vi "Autonomous Independent_17Feb.vi"() -> ()   [LabVIEW 2012]
doc: "This VI is called when autonomous begins, and will automatically be terminated when autonomous ends. You can carry out timed or sensor driven robot movement independently without needing to return to the caller."
uses:
  Robot Global Data.vi
  <vilib>/Rock Robotics/WPI/Joystick/WPI_JoystickGetSetRefNum.vi
  <vilib>/Rock Robotics/WPI/RobotDrive/WPI_RobotDriveArcadeDrive_Standard(NoSaturation).vi
panel:
  out "Prime 3":i32
  out "Prime 2.1":i32
  out "Prime 1.1":i32
  out "Prime 2":i32
  out "Prime 1":i32
  out "Report 2":i32
  out "Report 1":i32
  out "Count 3":bool
  out "Count 2":bool
  out "Count 1":bool
  out "S3":i32
  out "S2":i32
  out "S1":i32
  in  "Auton Pitch":dbl=30.5
  in  "Auton RPM":dbl=4200.0
  in  "milliseconds to wait\nduring autonomous":u32
  in  "Desired angle to\nturn to align with feeder\nstation 2":dbl
  in  "Desired distance for\nencoder to travel straight\ntowards wall 2":dbl
  in  "Desired angle to\nturn towards wall 2":dbl
  in  "Desired distance for\nthe encoder to count 2":dbl
  in  "Desired angle to turn\nBackwards (180) 2":dbl
  in  "Autonomous Modes":T1(ring)
  in  "Desired angle to\nturn to align with feeder\nstation":dbl
  in  "Desired distance for\nencoder to travel straight\ntowards wall":dbl
  in  "Desired angle to\nturn towards wall":dbl
  in  "Desired distance for\nthe encoder to count":dbl
  in  "Desired angle to turn\nBackwards (180)":dbl
  out "Current Movement, for debugging":T2 {"Y Joystick Value" scale=1.0..-1.0; "X Joystick Value" scale=-1.0..1.0}
  in  "Array of robot movements":T3(array[cluster]) {"Y Joystick Value" scale=1.0..-1.0; "X Joystick Value" scale=-1.0..1.0}
  # "Pre-Shot"
  # "Shoot 1"
  # "Shoot 2"
  # "To Align With Protected Feeder Station"
  # "To Align With Unprotected Feeder Station"
  # "Shoot 3"
  # "Be sure to right-click and choose Data Operations>>Make Current Value default if you want to save the array values with the VI"
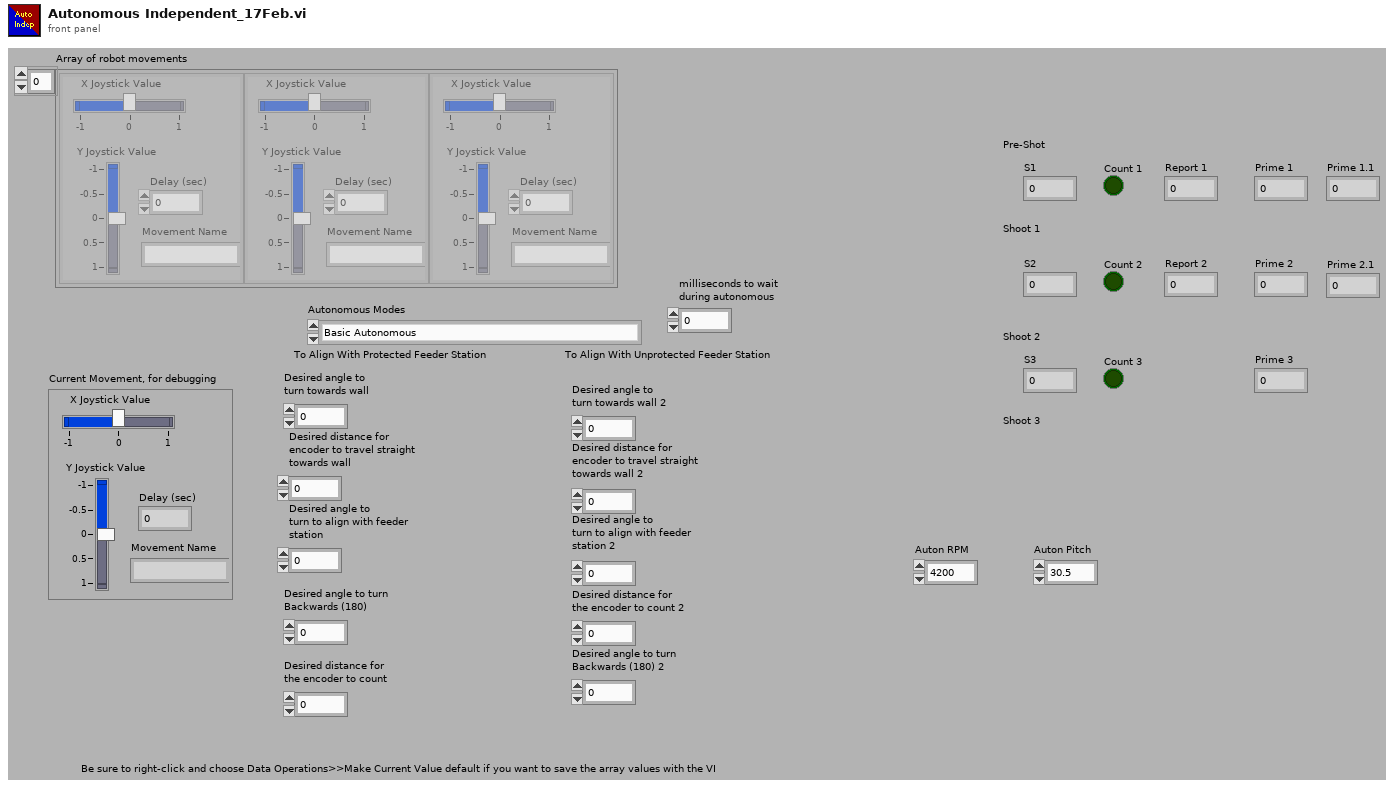
[diagram p1: front panel]
types:
  T1 = enum16{"Basic Autonomous", "Delayed Autonomous", "Shoot and Line Up With Protected Feeder Station", "Shoot and Line Up With Unprotected Feeder Station"}
  T2 = cluster{"X Joystick Value":dbl, "Y Joystick Value":dbl, "Delay (sec)":dbl, "Movement Name":string}
  T3 = cluster{"X Joystick Value":dbl, "Y Joystick Value":dbl, "Delay (sec)":dbl, "Movement Name":string}[]
  T4 = typedef "WPI_JoystickDevRef.ctl" = cluster{"Device":T5}
  T5 = typedef "WPI_JoystickDeviceEnum.ctl" = enum16{"USB 1", "USB 2", "USB 3", "USB 4", "Kinect 1", "Kinect 2"}
  T6 = cluster{"axis 1 (x)":dbl, "axis 2 (y)":dbl, "axis 3 (throttle)":dbl, "axis 4":dbl, "axis 5":dbl, "axis 6":dbl}
  T7 = typedef "WPI_RobotDriveDevRef.ctl" = cluster{"DevStatus":errorcluster, "Motors[]":T8[], "Square Inputs":bool, "Max Output":dbl, "Isochronous":bool}
  T8 = typedef "WPI_MotorControlDeviceRef.ctl" = cluster{"DeviceStatus":errorcluster, "Type":enum16{"PWM", "CAN"}, "PWM":cluster{"Digital Module":T9, "PWM Channel":T10, "DeadBand":T11}, "CAN":cluster{"Device Number":u8, "Control Mode":T12, "Semaphore":T13, "Max Vout":dbl}, "Invert":bool, "TransformRef":T14, "InvTransformRef":T14}
  T9 = typedef "FPGA_TypedefDigitalModule.ctl" = enum16{"Digital Module 1", "Digital Module 2"}
  T10 = typedef "FPGA_DIOPWMChannel.ctl" = enum8{"PWM 1", "PWM 2", "PWM 3", "PWM 4", "PWM 5", "PWM 6", "PWM 7", "PWM 8", "PWM 9", "PWM 10", "Invalid"}
  T11 = typedef "WPI_PWMDeadband.ctl" = cluster{"Name":string, "maxPositivePwm":i32, "minPositivePwm":i32, "centerPwm":i32, "maxNegativePwm":i32, "minNegativePwm":i32, "angularRange":u16}
  T12 = typedef "WPI_CANJaguar_ControlMode.ctl" = enum8{"Percent VBus", "Current", "Speed", "Position", "Voltage"}
  T13 = typedef "Semaphore RefNum" = refnum<k1>
  T14 = typedef "WPI_PWMTransform_ConPane.ctl" = refnum<vi>
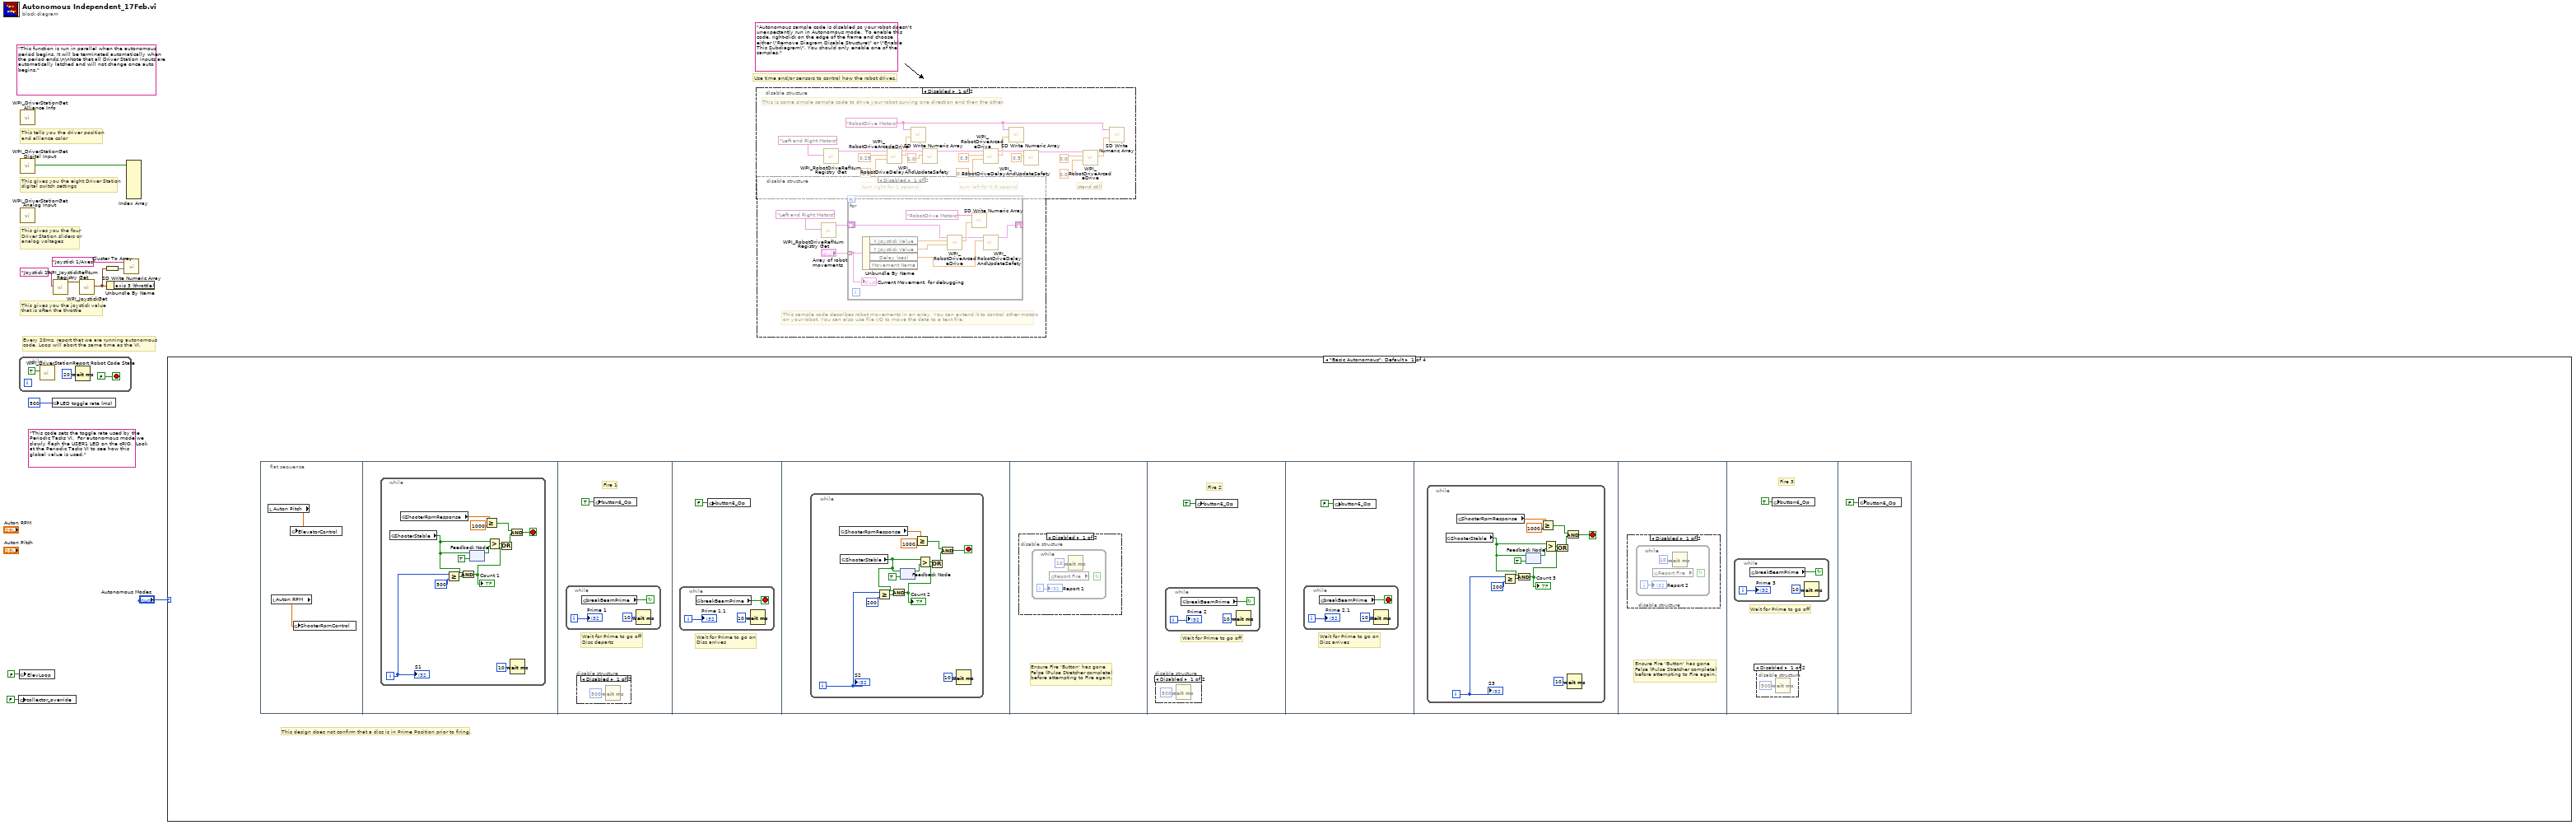
[diagram p0: block diagram]
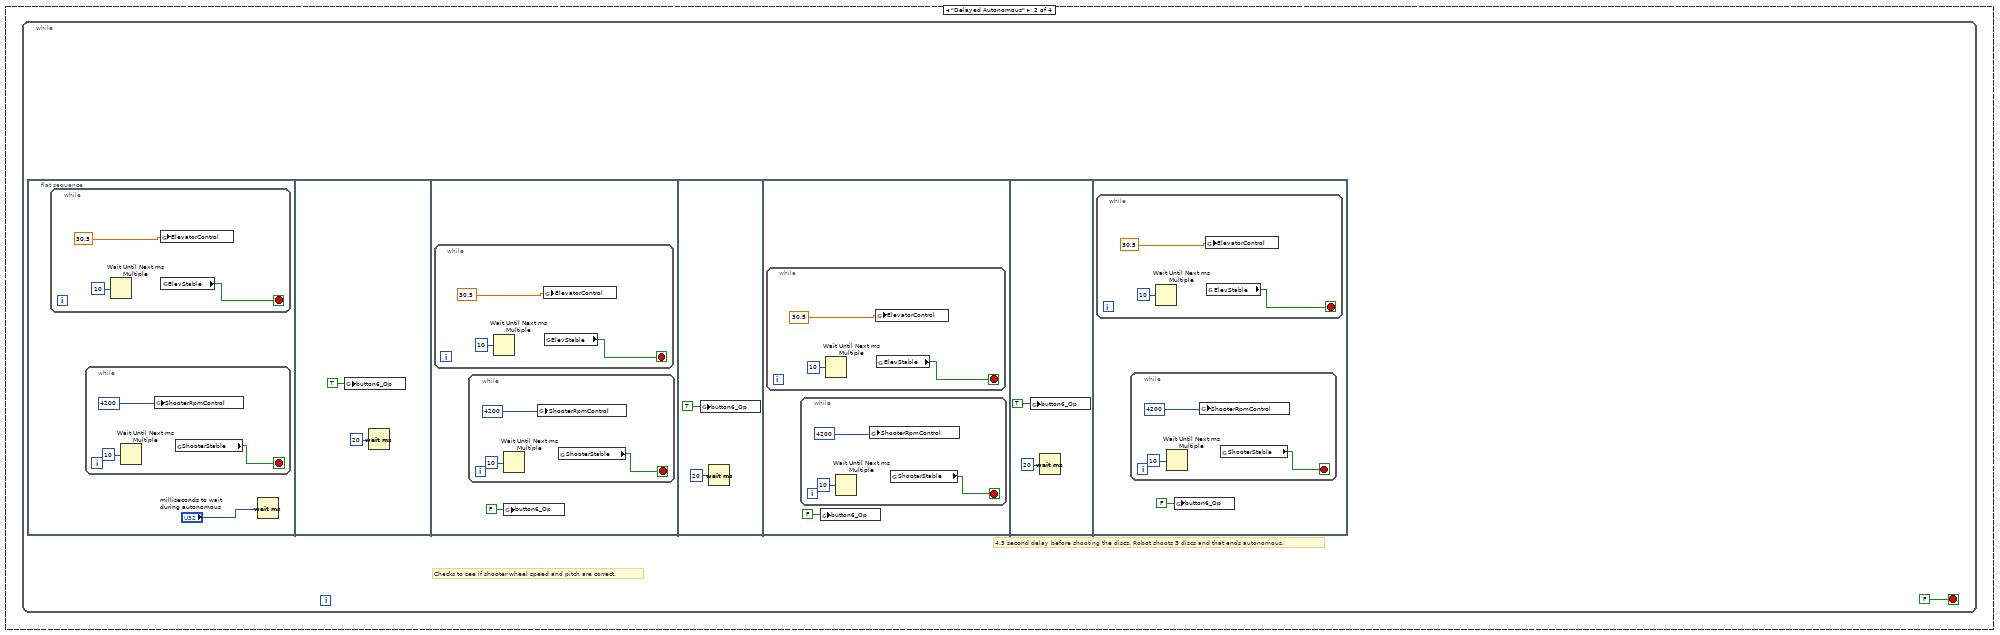
[diagram p7: hidden frame]
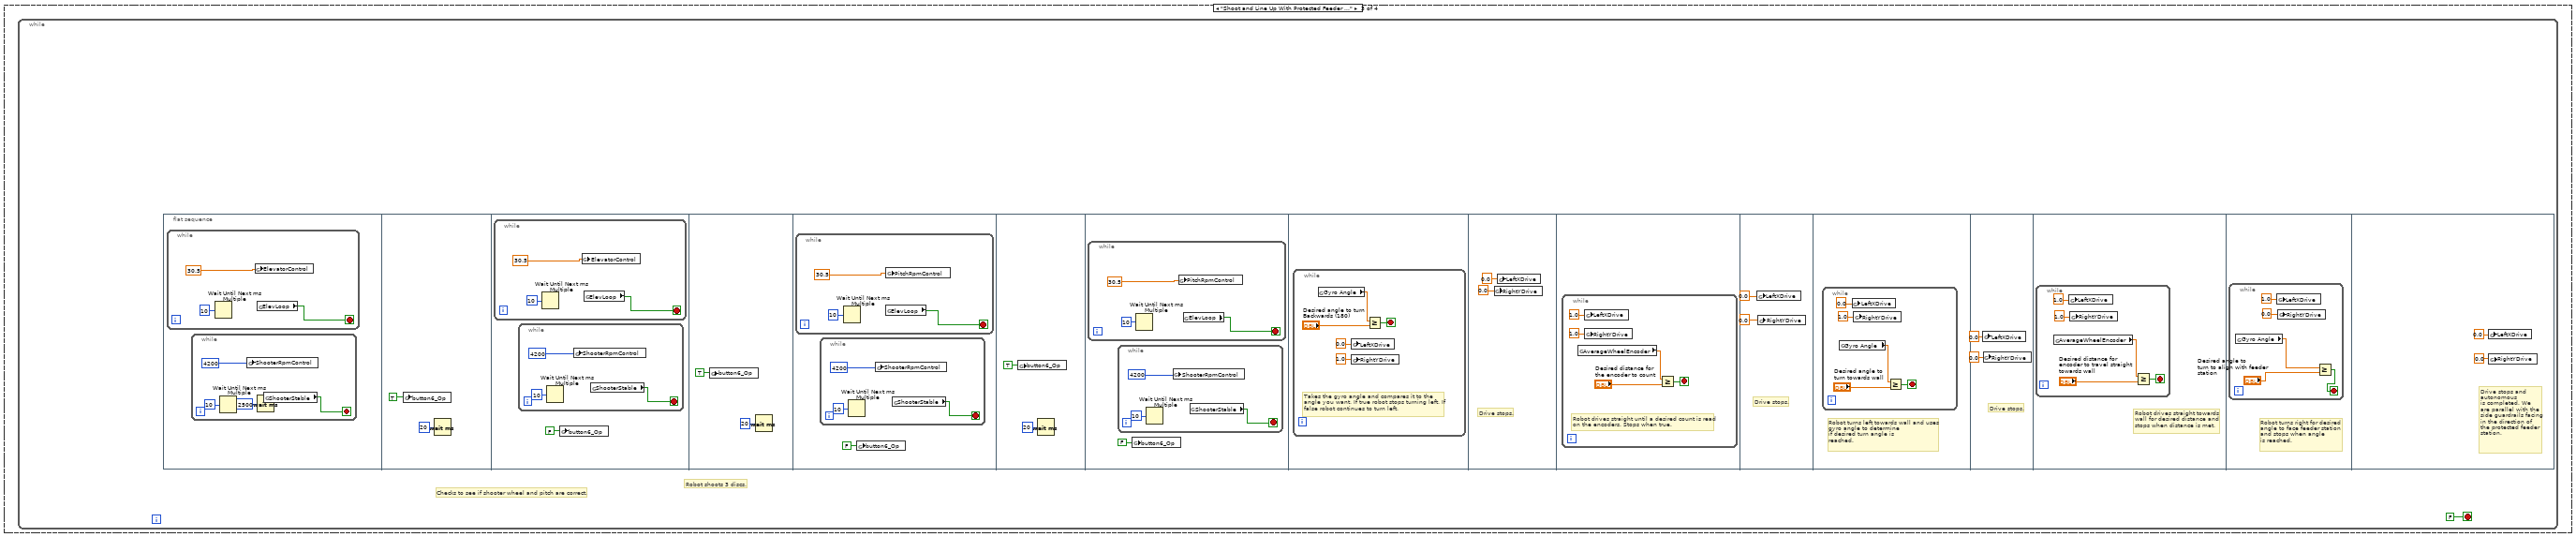
[diagram p8: hidden frame]
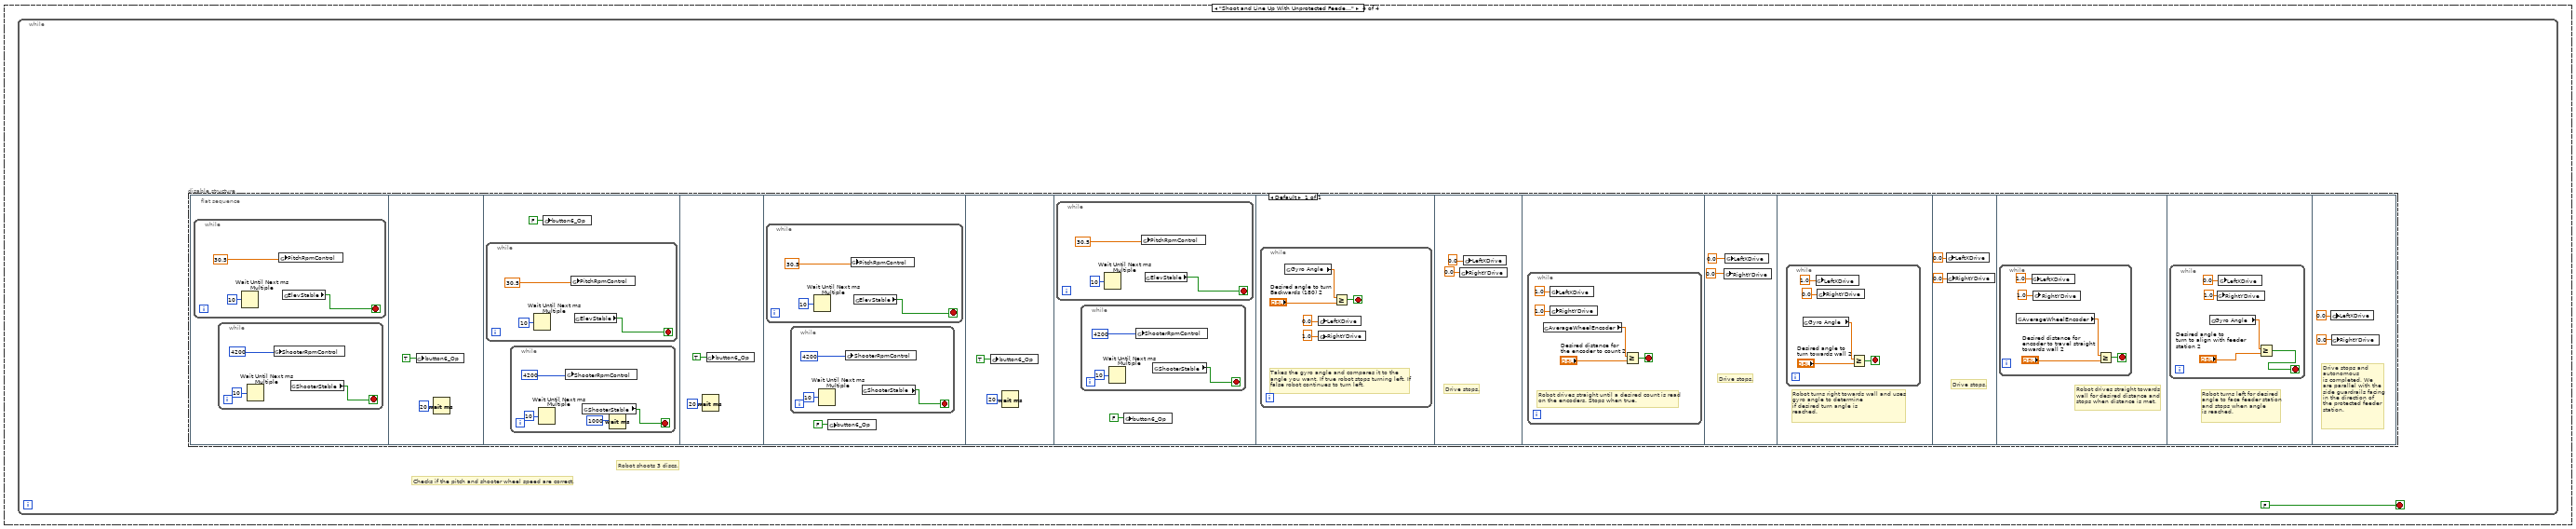
[diagram p9: hidden frame]
diagram:
  (unwired) "This code sets the toggle rate used by the Periodic Tasks VI.  For autonomous mode we slowly flash the USER1 LED on the cRIO.  Look at the Periodic Tasks VI to see how this global value is used."
  (unwired) "Autonomous sample code is disabled so your robot doesn't unexpectantly run in Autonomous mode.  To enable this code, right-click on the edge of the frame and choose either \"Remove Diagram Disable Structure\" or \"Enable This Subdiagram\". You should only enable one of the samples."
  (unwired) "This function is run in parallel when the autonomous period begins. It will be terminated automatically when the period ends.\n\nNote that all Driver Station inputs are automatically latched and will not change once auto begins."
  # "Every 20ms, report that we are running autonomous\ncode. Loop will abort the same time as the VI."
  # "This gives you the joystick value\nthat is often the throttle"
  # "Use time and/or sensors to control how the robot drives."
  # "This tells you the driver position\nand alliance color"
  # "This gives you the eight Driver Station\ndigital switch settings"
  # "This gives you the four\nDriver Station sliders or\nanalog voltages"
  n1 = global write "Robot Global Data.vi" "collector_override"(FALSE ("collector_override")) -> ()
  n2 = global write "Robot Global Data.vi" "ElevLoop"(FALSE ("ElevLoop")) -> ()
  n3 = while {
    stop <- FALSE stop-if-true
    n4 = call <vilib>:"WPI_DriverStationReport Robot Code State.vi"("Autonomous"=TRUE) -> ()  [unwired: 10 in, 1 out]
    n5 = Wait (ms)(milliseconds to wait=u32 20) -> ()  [unwired: 1 out]
  }
  n6 = call <vilib>:"WPI_DriverStationGet Alliance Info.vi"() -> ()  [unwired: 12 out]
  n7 = call <vilib>:"WPI_DriverStationGet Digital Input.vi"() -> ("Driver Station Digital Input (1-8)"=w10:bool[])  [unwired: 11 out]
  n8 = call <vilib>:"WPI_DriverStationGet Analog Input.vi"() -> ()  [unwired: 12 out]
  n9 = global write "Robot Global Data.vi" "LED toggle rate (ms)"(u32 500 ("LED ms toggle rate")) -> ()
  n10 = call <vilib>:"WPI_JoystickRefNum Registry Get.vi"("refnum name"="Joystick 1") -> ("JoystickDevRef"=w8:T4)  [unwired: 1 in, 9 out]
  n11 = call <vilib>:"WPI_JoystickGet.vi"("JoystickDevRef"=w8) -> ("Axes"=w5:T6)  [unwired: 1 in, 5 out]
  n12 = Cluster To Array(cluster=w5) -> (array=w6:dbl[])
  n13 = Unbundle By Name(w5) -> ()  [unwired: 1 out]
  n14 = call <vilib>:"SD Write Numeric Array.vi"("Numeric Array"=w6, "Name"="Joystick 1/Axes") -> ()  [unwired: 8 in, 2 out]
  n15 = Index Array(array=w10) -> ()  [unwired: 8 in, 8 out]
  n16 = case shown="\"Basic Autonomous\", Default" "Autonomous Modes" {
    frame "Basic Autonomous", Default {
      # "This design does not confirm that a disc is in Prime Position prior to firing."
      n17 = flat-sequence {
        frame #0 {
          n18 = local read "Auton Pitch"() -> (w15:dbl)
          n19 = local read "Auton RPM"() -> (w14:dbl)
          n20 = global write "Robot Global Data.vi" "ElevatorControl"(w15) -> ()
          n21 = global write "Robot Global Data.vi" "ShooterRpmControl"(w14) -> ()
        }
        frame #1 {
          n22 = while {
            i -> [w18]
            stop <- w16 stop-if-true
            n23 = global read "Robot Global Data.vi" "ShooterStable"() -> (w17:bool)
            n24 = global read "Robot Global Data.vi" "ShooterRpmResponse"() -> (w19:dbl)
            n25 = Greater Or Equal?(x=w18, y=500) -> (x >= y?=w24:bool)
            n26 = And(x=w17, y=w24) -> (x .and. y?=w26:bool)
            "Count 1" <- w26
            n27 = feedback #1(TRUE ("Shooter Stable?")) -> (w22:bool)
            n28 = feedback-in #1(w17) -> ()
            n29 = Greater Or Equal?(x=w19, y=1000.0) -> (x >= y?=w21:bool)
            n30 = Greater?(x=w17, y=w22) -> (0:w27:bool)
            n31 = Or(x=w27, y=w26) -> (x .or. y?=w28:bool)
            n32 = And(x=w21, y=w28) -> (x .and. y?=w16:bool)
            n33 = Wait (ms)(milliseconds to wait=u32 10 ("millisecond multiple")) -> ()  [unwired: 1 out]
            "S1" <- w18
          }
        }
        frame #2 {
          # "Wait for Prime to go off\nDisc departs"
          # "Fire 1"
          n34 = while {
            i -> [w32]
            stop <- w34 continue-if-true
            n35 = global read "Robot Global Data.vi" "breakBeamPrime"() -> (w34:bool)
            n36 = Wait (ms)(milliseconds to wait=u32 10 ("millisecond multiple")) -> ()  [unwired: 1 out]
            "Prime 1" <- w32
          }
          n37 = disable-structure shown="Disabled" {
            frame Disabled {
              n38 = Wait (ms)(milliseconds to wait=u32 500) -> ()  [unwired: 1 out]
            }
            frame Enabled {
            }
          }
          n39 = global write "Robot Global Data.vi" "button6_Op"(TRUE ("button5_Op")) -> ()
        }
        frame #3 {
          # "Wait for Prime to go on\nDisc arrives"
          n40 = while {
            i -> [w36]
            stop <- w38 stop-if-true
            n41 = global read "Robot Global Data.vi" "breakBeamPrime"() -> (w38:bool)
            n42 = Wait (ms)(milliseconds to wait=u32 10 ("millisecond multiple")) -> ()  [unwired: 1 out]
            "Prime 1.1" <- w36
          }
          n43 = global write "Robot Global Data.vi" "button6_Op"(FALSE ("button5_Op")) -> ()
        }
        frame #4 {
          n44 = while {
            i -> [w40]
            stop <- w39 stop-if-true
            n45 = global read "Robot Global Data.vi" "ShooterRpmResponse"() -> (w51:dbl)
            n46 = global read "Robot Global Data.vi" "ShooterStable"() -> (w43:bool)
            n47 = Greater Or Equal?(x=w40, y=200) -> (x >= y?=w46:bool)
            n48 = And(x=w43, y=w46) -> (x .and. y?=w44:bool)
            "Count 2" <- w44
            n49 = feedback #2(TRUE ("Shooter Stable?")) -> (w48:bool)
            n50 = feedback-in #2(w43) -> ()
            n51 = Greater Or Equal?(x=w51, y=1000.0) -> (x >= y?=w49:bool)
            n52 = Greater?(x=w43, y=w48) -> (0:w42:bool)
            n53 = Or(x=w42, y=w44) -> (x .or. y?=w41:bool)
            n54 = And(x=w49, y=w41) -> (x .and. y?=w39:bool)
            n55 = Wait (ms)(milliseconds to wait=u32 10 ("millisecond multiple")) -> ()  [unwired: 1 out]
            "S2" <- w40
          }
        }
        frame #5 {
          # "Ensure Fire 'Button' has gone\nFalse (Pulse Stretcher complete)\nbefore attempting to Fire again."
          n56 = disable-structure shown="Disabled" {
            frame Disabled {
              n57 = while {
                i -> [w54]
                stop <- _ continue-if-true
                n58 = global read "Robot Global Data.vi" "Report Fire"() -> ()  [unwired: 1 out]
                n59 = Wait (ms)(milliseconds to wait=u32 10) -> ()  [unwired: 1 out]
                "Report 1" <- w54
              }
            }
            frame Enabled {
            }
          }
        }
        frame #6 {
          # "Wait for Prime to go off"
          # "Fire 2"
          n60 = disable-structure shown="Disabled" {
            frame Disabled {
              n61 = Wait (ms)(milliseconds to wait=u32 500) -> ()  [unwired: 1 out]
            }
            frame Enabled {
            }
          }
          n62 = while {
            i -> [w56]
            stop <- w58 continue-if-true
            n63 = global read "Robot Global Data.vi" "breakBeamPrime"() -> (w58:bool)
            n64 = Wait (ms)(milliseconds to wait=u32 10 ("millisecond multiple")) -> ()  [unwired: 1 out]
            "Prime 2" <- w56
          }
          n65 = global write "Robot Global Data.vi" "button6_Op"(TRUE ("button5_Op")) -> ()
        }
        frame #7 {
          # "Wait for Prime to go on\nDisc arrives"
          n66 = while {
            i -> [w61]
            stop <- w63 stop-if-true
            n67 = global read "Robot Global Data.vi" "breakBeamPrime"() -> (w63:bool)
            n68 = Wait (ms)(milliseconds to wait=u32 10 ("millisecond multiple")) -> ()  [unwired: 1 out]
            "Prime 2.1" <- w61
          }
          n69 = global write "Robot Global Data.vi" "button6_Op"(FALSE ("button5_Op")) -> ()
        }
        frame #8 {
          n70 = while {
            i -> [w65]
            stop <- w64 stop-if-true
            n71 = global read "Robot Global Data.vi" "ShooterStable"() -> (w66:bool)
            n72 = global read "Robot Global Data.vi" "ShooterRpmResponse"() -> (w67:dbl)
            n73 = Greater Or Equal?(x=w65, y=200) -> (x >= y?=w72:bool)
            n74 = And(x=w66, y=w72) -> (x .and. y?=w74:bool)
            "Count 3" <- w74
            n75 = feedback #3(TRUE ("Shooter Stable?")) -> (w70:bool)
            n76 = feedback-in #3(w66) -> ()
            n77 = Greater Or Equal?(x=w67, y=1000.0) -> (x >= y?=w69:bool)
            n78 = Greater?(x=w66, y=w70) -> (0:w75:bool)
            n79 = Or(x=w75, y=w74) -> (x .or. y?=w76:bool)
            n80 = And(x=w69, y=w76) -> (x .and. y?=w64:bool)
            n81 = Wait (ms)(milliseconds to wait=u32 10 ("millisecond multiple")) -> ()  [unwired: 1 out]
            "S3" <- w65
          }
        }
        frame #9 {
          # "Ensure Fire 'Button' has gone\nFalse (Pulse Stretcher complete)\nbefore attempting to Fire again."
          n82 = disable-structure shown="Disabled" {
            frame Disabled {
              n83 = while {
                i -> [w79]
                stop <- _ continue-if-true
                n84 = global read "Robot Global Data.vi" "Report Fire"() -> ()  [unwired: 1 out]
                n85 = Wait (ms)(milliseconds to wait=u32 10) -> ()  [unwired: 1 out]
                "Report 2" <- w79
              }
            }
            frame Enabled {
            }
          }
        }
        frame #10 {
          # "Wait for Prime to go off"
          # "Fire 3"
          n86 = while {
            i -> [w81]
            stop <- w83 continue-if-true
            n87 = global read "Robot Global Data.vi" "breakBeamPrime"() -> (w83:bool)
            n88 = Wait (ms)(milliseconds to wait=u32 10 ("millisecond multiple")) -> ()  [unwired: 1 out]
            "Prime 3" <- w81
          }
          n89 = disable-structure shown="Disabled" {
            frame Disabled {
              n90 = Wait (ms)(milliseconds to wait=u32 500) -> ()  [unwired: 1 out]
            }
            frame Enabled {
            }
          }
          n91 = global write "Robot Global Data.vi" "button6_Op"(TRUE ("button5_Op")) -> ()
        }
        frame #11 {
          n92 = global write "Robot Global Data.vi" "button6_Op"(FALSE ("button5_Op")) -> ()
        }
      }
    }
    frame "Delayed Autonomous" {
      n93 = while {
        stop <- FALSE stop-if-true
        # "Checks to see if shooter wheel speed and pitch are correct."
        # "4.5 second delay before shooting the discs. Robot shoots 3 discs and that ends autonomous."
        n94 = flat-sequence {
          frame #0 {
            n95 = while {
              stop <- w89 stop-if-true
              n96 = Wait Until Next ms Multiple(millisecond multiple=u32 10) -> ()  [unwired: 1 out]
              n97 = global write "Robot Global Data.vi" "ElevatorControl"(30.5 ("y")) -> ()
              n98 = global read "Robot Global Data.vi" "ElevStable"() -> (w89:bool)
            }
            n99 = while {
              stop <- w92 stop-if-true
              n100 = Wait Until Next ms Multiple(millisecond multiple=u32 10) -> ()  [unwired: 1 out]
              n101 = global write "Robot Global Data.vi" "ShooterRpmControl"(4200 ("Value")) -> ()
              n102 = global read "Robot Global Data.vi" "ShooterStable"() -> (w92:bool)
            }
            n103 = Wait (ms)(milliseconds to wait="milliseconds to wait\nduring autonomous") -> ()  [unwired: 1 out]
          }
          frame #1 {
            n104 = global write "Robot Global Data.vi" "button6_Op"(TRUE ("button5_Op")) -> ()
            n105 = Wait (ms)(milliseconds to wait=u32 20) -> ()  [unwired: 1 out]
          }
          frame #2 {
            n106 = while {
              stop <- w98 stop-if-true
              n107 = Wait Until Next ms Multiple(millisecond multiple=u32 10) -> ()  [unwired: 1 out]
              n108 = global write "Robot Global Data.vi" "ElevatorControl"(30.5 ("y")) -> ()
              n109 = global read "Robot Global Data.vi" "ElevStable"() -> (w98:bool)
            }
            n110 = while {
              stop <- w101 stop-if-true
              n111 = Wait Until Next ms Multiple(millisecond multiple=u32 10) -> ()  [unwired: 1 out]
              n112 = global write "Robot Global Data.vi" "ShooterRpmControl"(4200 ("Value")) -> ()
              n113 = global read "Robot Global Data.vi" "ShooterStable"() -> (w101:bool)
            }
            n114 = global write "Robot Global Data.vi" "button6_Op"(FALSE ("button5_Op")) -> ()
          }
          frame #3 {
            n115 = global write "Robot Global Data.vi" "button6_Op"(TRUE ("button5_Op")) -> ()
            n116 = Wait (ms)(milliseconds to wait=u32 20) -> ()  [unwired: 1 out]
          }
          frame #4 {
            n117 = while {
              stop <- w107 stop-if-true
              n118 = Wait Until Next ms Multiple(millisecond multiple=u32 10) -> ()  [unwired: 1 out]
              n119 = global write "Robot Global Data.vi" "ElevatorControl"(30.5 ("y")) -> ()
              n120 = global read "Robot Global Data.vi" "ElevStable"() -> (w107:bool)
            }
            n121 = while {
              stop <- w110 stop-if-true
              n122 = Wait Until Next ms Multiple(millisecond multiple=u32 10) -> ()  [unwired: 1 out]
              n123 = global write "Robot Global Data.vi" "ShooterRpmControl"(4200 ("Value")) -> ()
              n124 = global read "Robot Global Data.vi" "ShooterStable"() -> (w110:bool)
            }
            n125 = global write "Robot Global Data.vi" "button6_Op"(FALSE ("button5_Op")) -> ()
          }
          frame #5 {
            n126 = global write "Robot Global Data.vi" "button6_Op"(TRUE ("button5_Op")) -> ()
            n127 = Wait (ms)(milliseconds to wait=u32 20) -> ()  [unwired: 1 out]
          }
          frame #6 {
            n128 = while {
              stop <- w116 stop-if-true
              n129 = Wait Until Next ms Multiple(millisecond multiple=u32 10) -> ()  [unwired: 1 out]
              n130 = global write "Robot Global Data.vi" "ElevatorControl"(30.5 ("y")) -> ()
              n131 = global read "Robot Global Data.vi" "ElevStable"() -> (w116:bool)
            }
            n132 = while {
              stop <- w119 stop-if-true
              n133 = Wait Until Next ms Multiple(millisecond multiple=u32 10) -> ()  [unwired: 1 out]
              n134 = global write "Robot Global Data.vi" "ShooterRpmControl"(4200 ("Value")) -> ()
              n135 = global read "Robot Global Data.vi" "ShooterStable"() -> (w119:bool)
            }
            n136 = global write "Robot Global Data.vi" "button6_Op"(FALSE ("button5_Op")) -> ()
          }
        }
      }
    }
    frame "Shoot and Line Up With Protected Feeder Station" {
      n137 = while {
        stop <- FALSE stop-if-true
        # "Checks to see if shooter wheel and pitch are correct."
        # "Robot shoots 3 discs."
        n138 = flat-sequence {
          frame #0 {
            n139 = while {
              stop <- w124 stop-if-true
              n140 = Wait Until Next ms Multiple(millisecond multiple=u32 10) -> ()  [unwired: 1 out]
              n141 = global write "Robot Global Data.vi" "ElevatorControl"(30.5 ("y")) -> ()
              n142 = global read "Robot Global Data.vi" "ElevLoop"() -> (w124:bool)
            }
            n143 = while {
              stop <- w127 stop-if-true
              n144 = Wait Until Next ms Multiple(millisecond multiple=u32 10) -> ()  [unwired: 1 out]
              n145 = global write "Robot Global Data.vi" "ShooterRpmControl"(4200 ("Value")) -> ()
              n146 = global read "Robot Global Data.vi" "ShooterStable"() -> (w127:bool)
            }
            n147 = Wait (ms)(milliseconds to wait=u32 2500) -> ()  [unwired: 1 out]
          }
          frame #1 {
            n148 = global write "Robot Global Data.vi" "button6_Op"(TRUE ("button5_Op")) -> ()
            n149 = Wait (ms)(milliseconds to wait=u32 20) -> ()  [unwired: 1 out]
          }
          frame #2 {
            n150 = while {
              stop <- w133 stop-if-true
              n151 = Wait Until Next ms Multiple(millisecond multiple=u32 10) -> ()  [unwired: 1 out]
              n152 = global write "Robot Global Data.vi" "ElevatorControl"(30.5 ("y")) -> ()
              n153 = global read "Robot Global Data.vi" "ElevLoop"() -> (w133:bool)
            }
            n154 = while {
              stop <- w136 stop-if-true
              n155 = Wait Until Next ms Multiple(millisecond multiple=u32 10) -> ()  [unwired: 1 out]
              n156 = global write "Robot Global Data.vi" "ShooterRpmControl"(4200 ("Value")) -> ()
              n157 = global read "Robot Global Data.vi" "ShooterStable"() -> (w136:bool)
            }
            n158 = global write "Robot Global Data.vi" "button6_Op"(FALSE ("button5_Op")) -> ()
          }
          frame #3 {
            n159 = global write "Robot Global Data.vi" "button6_Op"(TRUE ("button5_Op")) -> ()
            n160 = Wait (ms)(milliseconds to wait=u32 20) -> ()  [unwired: 1 out]
          }
          frame #4 {
            n161 = while {
              stop <- w142 stop-if-true
              n162 = Wait Until Next ms Multiple(millisecond multiple=u32 10) -> ()  [unwired: 1 out]
              n163 = global read "Robot Global Data.vi" "ElevLoop"() -> (w142:bool)
              n164 = global write "Robot Global Data.vi" "PitchRpmControl"(30.5 ("y")) -> ()
            }
            n165 = while {
              stop <- w145 stop-if-true
              n166 = Wait Until Next ms Multiple(millisecond multiple=u32 10) -> ()  [unwired: 1 out]
              n167 = global write "Robot Global Data.vi" "ShooterRpmControl"(4200 ("Value")) -> ()
              n168 = global read "Robot Global Data.vi" "ShooterStable"() -> (w145:bool)
            }
            n169 = global write "Robot Global Data.vi" "button6_Op"(FALSE ("button5_Op")) -> ()
          }
          frame #5 {
            n170 = global write "Robot Global Data.vi" "button6_Op"(TRUE ("button5_Op")) -> ()
            n171 = Wait (ms)(milliseconds to wait=u32 20) -> ()  [unwired: 1 out]
          }
          frame #6 {
            n172 = while {
              stop <- w151 stop-if-true
              n173 = Wait Until Next ms Multiple(millisecond multiple=u32 10) -> ()  [unwired: 1 out]
              n174 = global write "Robot Global Data.vi" "PitchRpmControl"(30.5 ("y")) -> ()
              n175 = global read "Robot Global Data.vi" "ElevLoop"() -> (w151:bool)
            }
            n176 = while {
              stop <- w154 stop-if-true
              n177 = Wait Until Next ms Multiple(millisecond multiple=u32 10) -> ()  [unwired: 1 out]
              n178 = global write "Robot Global Data.vi" "ShooterRpmControl"(4200 ("Value")) -> ()
              n179 = global read "Robot Global Data.vi" "ShooterStable"() -> (w154:bool)
            }
            n180 = global write "Robot Global Data.vi" "button6_Op"(FALSE ("button5_Op")) -> ()
          }
          frame #7 {
            n181 = while {
              stop <- w160 stop-if-true
              # "Takes the gyro angle and compares it to the\nangle you want. If true robot stops turning left. If\nfalse robot continues to turn left."
              n182 = global read "Robot Global Data.vi" "Gyro Angle"() -> (w156:dbl)
              n183 = global write "Robot Global Data.vi" "LeftXDrive"(0.0 ("Left axis value")) -> ()
              n184 = global write "Robot Global Data.vi" "RightYDrive"(1.0 ("Right axis value")) -> ()
              n185 = Greater Or Equal?(x=w156, y="Desired angle to turn\nBackwards (180)") -> (x >= y?=w160:bool)
            }
          }
          frame #8 {
            # "Drive stops."
            n186 = global write "Robot Global Data.vi" "RightYDrive"(0.0 ("Right axis value")) -> ()
            n187 = global write "Robot Global Data.vi" "LeftXDrive"(0.0 ("Left axis value")) -> ()
          }
          frame #9 {
            n188 = while {
              stop <- w165 stop-if-true
              # "Robot drives straight until a desired count is read\non the encoders. Stops when true."
              n189 = global read "Robot Global Data.vi" "AverageWheelEncoder"() -> (w167:dbl)
              n190 = global write "Robot Global Data.vi" "LeftXDrive"(1.0 ("Left axis value")) -> ()
              n191 = global write "Robot Global Data.vi" "RightYDrive"(1.0 ("Right axis value")) -> ()
              n192 = Greater Or Equal?(x=w167, y="Desired distance for\nthe encoder to count") -> (x >= y?=w165:bool)
            }
          }
          frame #10 {
            # "Drive stops."
            n193 = global write "Robot Global Data.vi" "LeftXDrive"(0.0 ("LeftXDrive")) -> ()
            n194 = global write "Robot Global Data.vi" "RightYDrive"(0.0 ("LeftXDrive")) -> ()
          }
          frame #11 {
            # "Robot turns left towards wall and uses\ngyro angle to determine\nif desired turn angle is \nreached."
            n195 = while {
              stop <- w171 stop-if-true
              n196 = global read "Robot Global Data.vi" "Gyro Angle"() -> (w170:dbl)
              n197 = global write "Robot Global Data.vi" "LeftXDrive"(0.0 ("Left axis value")) -> ()
              n198 = global write "Robot Global Data.vi" "RightYDrive"(1.0 ("Right axis value")) -> ()
              n199 = Greater Or Equal?(x=w170, y="Desired angle to\nturn towards wall") -> (x >= y?=w171:bool)
            }
          }
          frame #12 {
            # "Drive stops."
            n200 = global write "Robot Global Data.vi" "LeftXDrive"(0.0 ("LeftXDrive")) -> ()
            n201 = global write "Robot Global Data.vi" "RightYDrive"(0.0 ("RightYDrive")) -> ()
          }
          frame #13 {
            # "Robot drives straight towards\nwall for desired distance and\nstops when distance is met."
            n202 = while {
              stop <- w177 stop-if-true
              n203 = global read "Robot Global Data.vi" "AverageWheelEncoder"() -> (w179:dbl)
              n204 = global write "Robot Global Data.vi" "LeftXDrive"(1.0 ("Left axis value")) -> ()
              n205 = global write "Robot Global Data.vi" "RightYDrive"(1.0 ("Right axis value")) -> ()
              n206 = Greater Or Equal?(x=w179, y="Desired distance for\nencoder to travel straight\ntowards wall") -> (x >= y?=w177:bool)
            }
          }
          frame #14 {
            # "Robot turns right for desired\nangle to face feeder station\nand stops when angle\nis reached."
            n207 = while {
              stop <- w183 stop-if-true
              n208 = global read "Robot Global Data.vi" "Gyro Angle"() -> (w182:dbl)
              n209 = global write "Robot Global Data.vi" "LeftXDrive"(1.0 ("Left axis value")) -> ()
              n210 = global write "Robot Global Data.vi" "RightYDrive"(0.0 ("Right axis value")) -> ()
              n211 = Greater Or Equal?(x=w182, y="Desired angle to\nturn to align with feeder\nstation") -> (x >= y?=w183:bool)
            }
          }
          frame #15 {
            # "Drive stops and\nautonomous\nis completed. We\nare parallel with the\nside guardrails facing\nin the direction of\nthe protected feeder\nstation."
            n212 = global write "Robot Global Data.vi" "LeftXDrive"(0.0 ("LeftXDrive")) -> ()
            n213 = global write "Robot Global Data.vi" "RightYDrive"(0.0 ("LeftXDrive")) -> ()
          }
        }
      }
    }
    frame "Shoot and Line Up With Unprotected Feeder Station" {
      n214 = while {
        stop <- FALSE stop-if-true
        # "Checks if the pitch and shooter wheel speed are correct."
        # "Robot shoots 3 discs."
        n215 = disable-structure shown="Default" {
          frame Enabled {
            n216 = flat-sequence {
              frame #0 {
                n217 = while {
                  stop <- w191 stop-if-true
                  n218 = Wait Until Next ms Multiple(millisecond multiple=u32 10) -> ()  [unwired: 1 out]
                  n219 = global write "Robot Global Data.vi" "PitchRpmControl"(30.5 ("y")) -> ()
                  n220 = global read "Robot Global Data.vi" "ElevStable"() -> (w191:bool)
                }
                n221 = while {
                  stop <- w194 stop-if-true
                  n222 = Wait Until Next ms Multiple(millisecond multiple=u32 10) -> ()  [unwired: 1 out]
                  n223 = global write "Robot Global Data.vi" "ShooterRpmControl"(4200 ("Value")) -> ()
                  n224 = global read "Robot Global Data.vi" "ShooterStable"() -> (w194:bool)
                }
              }
              frame #1 {
                n225 = global write "Robot Global Data.vi" "button6_Op"(TRUE ("button5_Op")) -> ()
                n226 = Wait (ms)(milliseconds to wait=u32 20) -> ()  [unwired: 1 out]
              }
              frame #2 {
                n227 = while {
                  stop <- w201 stop-if-true
                  n228 = Wait Until Next ms Multiple(millisecond multiple=u32 10) -> ()  [unwired: 1 out]
                  n229 = global write "Robot Global Data.vi" "PitchRpmControl"(30.5 ("y")) -> ()
                  n230 = global read "Robot Global Data.vi" "ElevStable"() -> (w201:bool)
                }
                n231 = while {
                  stop <- w204 stop-if-true
                  n232 = Wait Until Next ms Multiple(millisecond multiple=u32 10) -> ()  [unwired: 1 out]
                  n233 = global write "Robot Global Data.vi" "ShooterRpmControl"(4200 ("Value")) -> ()
                  n234 = global read "Robot Global Data.vi" "ShooterStable"() -> (w204:bool)
                }
                n235 = global write "Robot Global Data.vi" "button6_Op"(FALSE ("button5_Op")) -> ()
                n236 = Wait (ms)(milliseconds to wait=u32 1000) -> ()  [unwired: 1 out]
              }
              frame #3 {
                n237 = Wait (ms)(milliseconds to wait=u32 20) -> ()  [unwired: 1 out]
                n238 = global write "Robot Global Data.vi" "button6_Op"(TRUE ("button5_Op")) -> ()
              }
              frame #4 {
                n239 = while {
                  stop <- w210 stop-if-true
                  n240 = Wait Until Next ms Multiple(millisecond multiple=u32 10) -> ()  [unwired: 1 out]
                  n241 = global write "Robot Global Data.vi" "PitchRpmControl"(30.5 ("y")) -> ()
                  n242 = global read "Robot Global Data.vi" "ElevStable"() -> (w210:bool)
                }
                n243 = while {
                  stop <- w213 stop-if-true
                  n244 = Wait Until Next ms Multiple(millisecond multiple=u32 10) -> ()  [unwired: 1 out]
                  n245 = global write "Robot Global Data.vi" "ShooterRpmControl"(4200 ("Value")) -> ()
                  n246 = global read "Robot Global Data.vi" "ShooterStable"() -> (w213:bool)
                }
                n247 = global write "Robot Global Data.vi" "button6_Op"(FALSE ("button5_Op")) -> ()
              }
              frame #5 {
                n248 = global write "Robot Global Data.vi" "button6_Op"(TRUE ("button5_Op")) -> ()
                n249 = Wait (ms)(milliseconds to wait=u32 20) -> ()  [unwired: 1 out]
              }
              frame #6 {
                n250 = while {
                  stop <- w219 stop-if-true
                  n251 = Wait Until Next ms Multiple(millisecond multiple=u32 10) -> ()  [unwired: 1 out]
                  n252 = global write "Robot Global Data.vi" "PitchRpmControl"(30.5 ("y")) -> ()
                  n253 = global read "Robot Global Data.vi" "ElevStable"() -> (w219:bool)
                }
                n254 = while {
                  stop <- w222 stop-if-true
                  n255 = Wait Until Next ms Multiple(millisecond multiple=u32 10) -> ()  [unwired: 1 out]
                  n256 = global write "Robot Global Data.vi" "ShooterRpmControl"(4200 ("Value")) -> ()
                  n257 = global read "Robot Global Data.vi" "ShooterStable"() -> (w222:bool)
                }
                n258 = global write "Robot Global Data.vi" "button6_Op"(FALSE ("button5_Op")) -> ()
              }
              frame #7 {
                n259 = while {
                  stop <- w228 stop-if-true
                  # "Takes the gyro angle and compares it to the\nangle you want. If true robot stops turning left. If\nfalse robot continues to turn left."
                  n260 = global read "Robot Global Data.vi" "Gyro Angle"() -> (w224:dbl)
                  n261 = global write "Robot Global Data.vi" "LeftXDrive"(0.0 ("Left axis value")) -> ()
                  n262 = global write "Robot Global Data.vi" "RightYDrive"(1.0 ("Right axis value")) -> ()
                  n263 = Greater Or Equal?(x=w224, y="Desired angle to turn\nBackwards (180) 2") -> (x >= y?=w228:bool)
                }
              }
              frame #8 {
                # "Drive stops."
                n264 = global write "Robot Global Data.vi" "RightYDrive"(0.0 ("Right axis value")) -> ()
                n265 = global write "Robot Global Data.vi" "LeftXDrive"(0.0 ("Left axis value")) -> ()
              }
              frame #9 {
                n266 = while {
                  stop <- w233 stop-if-true
                  # "Robot drives straight until a desired count is read\non the encoders. Stops when true."
                  n267 = global read "Robot Global Data.vi" "AverageWheelEncoder"() -> (w235:dbl)
                  n268 = global write "Robot Global Data.vi" "LeftXDrive"(1.0 ("Left axis value")) -> ()
                  n269 = global write "Robot Global Data.vi" "RightYDrive"(1.0 ("Right axis value")) -> ()
                  n270 = Greater Or Equal?(x=w235, y="Desired distance for\nthe encoder to count 2") -> (x >= y?=w233:bool)
                }
              }
              frame #10 {
                # "Drive stops."
                n271 = global write "Robot Global Data.vi" "RightYDrive"(0.0 ("LeftXDrive")) -> ()
                n272 = global write "Robot Global Data.vi" "LeftXDrive"(0.0 ("LeftXDrive")) -> ()
              }
              frame #11 {
                # "Robot turns right towards wall and uses\ngyro angle to determine\nif desired turn angle is \nreached."
                n273 = while {
                  stop <- w239 stop-if-true
                  n274 = global read "Robot Global Data.vi" "Gyro Angle"() -> (w238:dbl)
                  n275 = global write "Robot Global Data.vi" "LeftXDrive"(1.0 ("Left axis value")) -> ()
                  n276 = global write "Robot Global Data.vi" "RightYDrive"(0.0 ("Right axis value")) -> ()
                  n277 = Greater Or Equal?(x=w238, y="Desired angle to\nturn towards wall 2") -> (x >= y?=w239:bool)
                }
              }
              frame #12 {
                # "Drive stops."
                n278 = global write "Robot Global Data.vi" "LeftXDrive"(0.0 ("LeftXDrive")) -> ()
                n279 = global write "Robot Global Data.vi" "RightYDrive"(0.0 ("RightYDrive")) -> ()
              }
              frame #13 {
                # "Robot drives straight towards\nwall for desired distance and\nstops when distance is met."
                n280 = while {
                  stop <- w245 stop-if-true
                  n281 = global read "Robot Global Data.vi" "AverageWheelEncoder"() -> (w247:dbl)
                  n282 = global write "Robot Global Data.vi" "LeftXDrive"(1.0 ("Left axis value")) -> ()
                  n283 = global write "Robot Global Data.vi" "RightYDrive"(1.0 ("Right axis value")) -> ()
                  n284 = Greater Or Equal?(x=w247, y="Desired distance for\nencoder to travel straight\ntowards wall 2") -> (x >= y?=w245:bool)
                }
              }
              frame #14 {
                # "Robot turns left for desired\nangle to face feeder station\nand stops when angle\nis reached."
                n285 = while {
                  stop <- w251 stop-if-true
                  n286 = global read "Robot Global Data.vi" "Gyro Angle"() -> (w250:dbl)
                  n287 = global write "Robot Global Data.vi" "RightYDrive"(1.0 ("Right axis value")) -> ()
                  n288 = global write "Robot Global Data.vi" "LeftXDrive"(0.0 ("Left axis value")) -> ()
                  n289 = Greater Or Equal?(x=w250, y="Desired angle to\nturn to align with feeder\nstation 2") -> (x >= y?=w251:bool)
                }
              }
              frame #15 {
                # "Drive stops and\nautonomous\nis completed. We\nare parallel with the\nside guardrails facing\nin the direction of\nthe protected feeder\nstation."
                n290 = global write "Robot Global Data.vi" "LeftXDrive"(0.0 ("LeftXDrive")) -> ()
                n291 = global write "Robot Global Data.vi" "RightYDrive"(0.0 ("LeftXDrive")) -> ()
              }
            }
          }
        }
      }
    }
  }
  n292 = disable-structure shown="Disabled" {
    frame Disabled {
      w257 = "RobotDrive Motors" ("Name")
      # "This is some simple sample code to drive your robot curving one direction and then the other."
      # "stand still"
      # "turn left for 0.5 second"
      # "turn right for 1 second"
      n293 = call <vilib>:"WPI_RobotDriveRefNum Registry Get.vi"("refnum name"="Left and Right Motors") -> ("RobotDriveDevRef"=w261:T7)  [unwired: 1 in, 9 out]
      n294 = call-poly <vilib>:"WPI_RobotDriveArcadeDrive.vi"("Y axis value"=0.5 ("X axis value"), "X axis value"=0.25, "RobotDriveDevRef"=w261) -> ("Motor Values"=w260:dbl[], "RobotDriveDevRef"=w268:T7)  [unwired: 1 in, 6 out]
      n295 = call <vilib>:"SD Write Numeric Array.vi"("Numeric Array"=w260, "Name"=w257) -> ()  [unwired: 8 in, 2 out]
      n296 = call <vilib>:"WPI_RobotDriveDelayAndUpdateSafety.vi"("Delay (s)"=1.0, "RobotDriveDevRef"=w268) -> ("RobotDriveDevRef 2"=w267:T7)  [unwired: 8 in, 1 out]
      n297 = call-poly <vilib>:"WPI_RobotDriveArcadeDrive.vi"("Y axis value"=0.25 ("X axis value"), "X axis value"=0.5, "RobotDriveDevRef"=w267) -> ("Motor Values"=w259:dbl[], "RobotDriveDevRef"=w266:T7)  [unwired: 1 in, 6 out]
      n298 = call <vilib>:"SD Write Numeric Array.vi"("Numeric Array"=w259, "Name"=w257) -> ()  [unwired: 8 in, 2 out]
      n299 = call <vilib>:"WPI_RobotDriveDelayAndUpdateSafety.vi"("Delay (s)"=0.5, "RobotDriveDevRef"=w266) -> ("RobotDriveDevRef 2"=w265:T7)  [unwired: 8 in, 1 out]
      n300 = call-poly <vilib>:"WPI_RobotDriveArcadeDrive.vi"("Y axis value"=0.0 ("X axis value"), "X axis value"=0.0, "RobotDriveDevRef"=w265) -> ("Motor Values"=w258:dbl[])  [unwired: 1 in, 7 out]
      n301 = call <vilib>:"SD Write Numeric Array.vi"("Numeric Array"=w258, "Name"=w257) -> ()  [unwired: 8 in, 2 out]
    }
    frame Enabled {
    }
  }
  n302 = disable-structure shown="Disabled" {
    frame Disabled {
      # "This sample code describes robot movements in an array. You can extend it to control other motors\non your robot. You can also use file I/O to move the data to a text file."
      n303 = call <vilib>:"WPI_RobotDriveRefNum Registry Get.vi"("refnum name"="Left and Right Motors") -> ("RobotDriveDevRef"=w276:T7)  [unwired: 1 in, 9 out]
      n304 = for {
        shift-right: [w282] -> _
        shift-left: w276 -> [w283]
        tunnel: "Array of robot movements" -> [w278] mode=indexing
        n305 = Unbundle By Name(w278) -> ("X Joystick Value"=w281:dbl, "Y Joystick Value"=w280:dbl, "Delay (sec)"=w279:dbl)  [unwired: 1 out]
        n306 = call-poly <vilib>:"WPI_RobotDriveArcadeDrive.vi"("Y axis value"=w280, "X axis value"=w281, "RobotDriveDevRef"=w283) -> ("Motor Values"=w285:dbl[], "RobotDriveDevRef"=w284:T7)  [unwired: 1 in, 6 out]
        n307 = call <vilib>:"SD Write Numeric Array.vi"("Numeric Array"=w285, "Name"="RobotDrive Motors") -> ()  [unwired: 8 in, 2 out]
        n308 = call <vilib>:"WPI_RobotDriveDelayAndUpdateSafety.vi"("Delay (s)"=w279, "RobotDriveDevRef"=w284) -> ("RobotDriveDevRef 2"=w282:T7)  [unwired: 8 in, 1 out]
        "Current Movement, for debugging" <- w278
      }
    }
    frame Enabled {
    }
  }
